vi "IStageGetPosition.vi"(5 "PRIORLib.IStageIn":refnum<k7>) -> (0 "YPos":dbl, 1 "XPos":dbl, 2 "error out":errorcluster, 3 "PRIORLib.IStageOut":refnum<k7>, 4 "Return":i32)   [LabVIEW 2011]
panel:
  # "This SubVi gets the stage position\nand returns immediately."
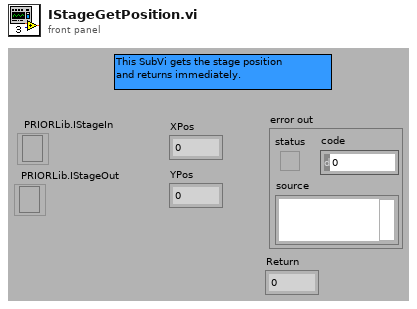
[diagram p1: front panel]
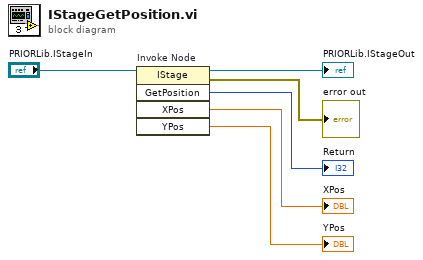
[diagram p0: block diagram]
diagram:
  n1 = invoke on="Invoke Node" class="IStage" method="GetPosition"(reference="PRIORLib.IStageIn") -> (reference out=→"PRIORLib.IStageOut":refnum<k7>, error out=→"error out":errorcluster, "GetPosition"=→"Return":i32, "XPos"=→"XPos":dbl, "YPos"=→"YPos":dbl)  [unwired: 4 in]
